vi "GUNSC_SetFunction.vi"(8 "error in (no error)":errorcluster, 10 "datatype":i32) -> (0 "error out":errorcluster, 2 "return value":i32)   [LabVIEW 2014]
uses:
  public/c/lib/libunsc.so
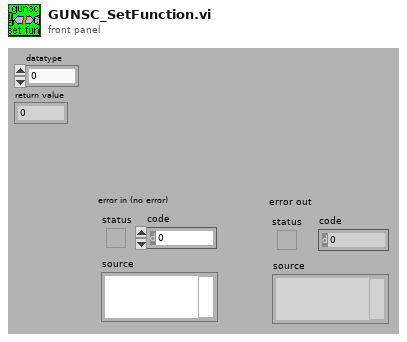
[diagram p1: front panel]
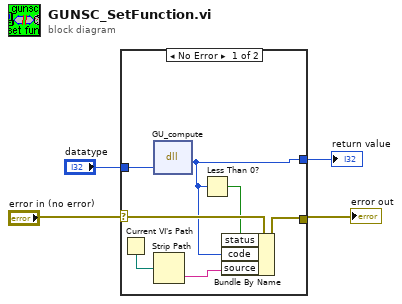
[diagram p0: block diagram]
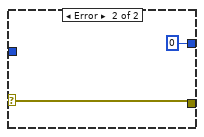
[diagram p2: hidden frame]
diagram:
  n1 = case shown="No Error" "error in (no error)" {
    selector: "error in (no error)" -> [w10 w13]
    tunnel: "datatype" -> [w11 _]
    tunnel: [w8 0] -> w3
    tunnel: [w5 w13] -> w1
    frame No Error {
      n2 = Current VI's Path() -> (path=w7:path)
      n3 = dll-call lib="home/sispi/Panview-1.13.0-64b/PAN/Modules/GUNSC/public/c/lib/libunsc.so" fn="GU_compute"("datatype"=w11) -> ("return type"=w8:i32)  [unwired: 4 in, 2 out]
      n4 = Strip Path(path=w7) -> (name=w6:string)  [unwired: 1 out]
      n5 = Less Than 0?(x=w8) -> (x < 0?=w9:bool)
      n6 = Bundle By Name(cluster=w10, "status"=w9, "code"=w8, "source"=w6) -> (w5:errorcluster)
    }
    frame Error {
    }
  }
  "return value" <- w3
  "error out" <- w1
